vi "ImageSetBaseOffset.vi"(8 "error in (no error)":errorcluster, 9 "channel":i32, 10 "offset":i32, 11 "Image in":refnum<class "Image.lvclass">) -> (0 "error out":errorcluster, 3 "Image out":refnum<class "Image.lvclass">)   [LabVIEW 2012, in "Image.lvclass"]
uses:
  classes/Image.lvclass
  classes/Image.lvclass/Image.ctl
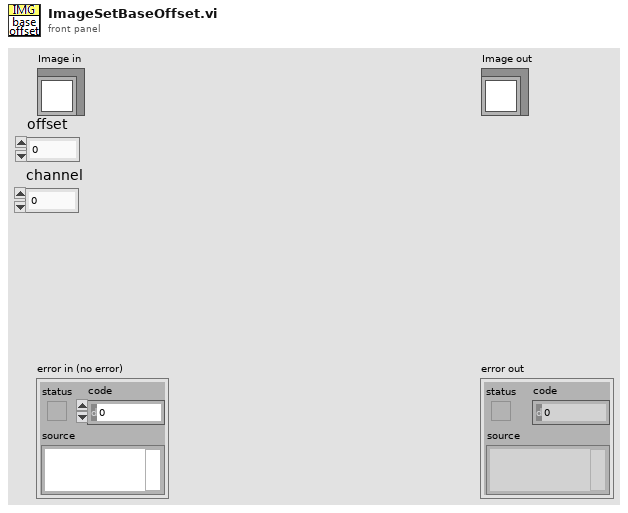
[diagram p1: front panel]
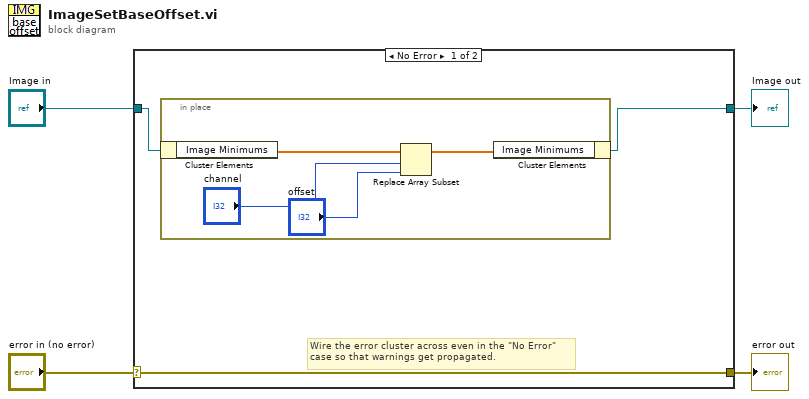
[diagram p0: block diagram]
diagram:
  n1 = case shown="No Error" "error in (no error)" {
    selector: "error in (no error)" -> [w7 w13]
    tunnel: [w7 w13] -> w3
    tunnel: [w5 w12] -> w1
    tunnel: "Image in" -> [w6 w12]
    frame No Error {
      # "Wire the error cluster across even in the \"No Error\"\ncase so that warnings get propagated."
      n2 = in-place {
        n3 = in-place-cluster #1(w6) -> ("Image Minimums"=w11:dbl[])
        n4 = Replace Array Subset(array=w11, new element="offset", index="channel") -> (w8:dbl[])
        n5 = in-place-cluster #1("Image Minimums"=w8) -> (w5:refnum<class "Image.lvclass">)
      }
    }
    frame Error {
    }
  }
  "error out" <- w3
  "Image out" <- w1
